vi "Cmd Get Parameter Properties (C).vi"(4 "error in (no error)":errorcluster, 6 "parameter index":variant, 7 "command reference":T4) -> (0 "error out":errorcluster, 1 "parameter properties":T1, 3 "command reference out":T4)   [LabVIEW 2017, in "NI_Database_API.lvlib"]
doc: "Gets properties of the object as determined by the inputs. This VI works for connections, commands, recordsets, columns, and parameters. Wire data to the reference input to determine the polymorphic instance to use or manually select the instance."
uses:
  <vilib>/addons/database/NI_Database_API.lvlib
  <vilib>/addons/database/Command.llb/Cmd ObjectReference.ctl
  <vilib>/addons/database/Command.llb/Cmd Parameter Properties.ctl
  <vilib>/addons/database/Auxilliary.llb/DB Tools DataTypes.ctl
  <vilib>/addons/database/Auxilliary.llb/DB Tools Parameter Dir.ctl
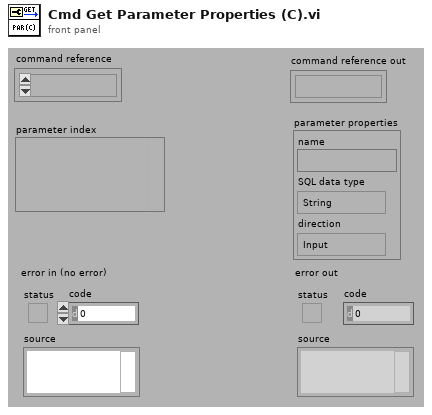
[diagram p1: front panel]
types:
  T1 = typedef "NI_Database_API.lvlib/Cmd Parameter Properties.ctl" = cluster{"name":string, "SQL data type":T2, "direction":T3}
  T2 = typedef "NI_Database_API.lvlib/DB Tools DataTypes.ctl" = enum16{"String", "Long (I32)", "Single (SGL)", "Double (DBL)", "Date/Time", "Binary"}
  T3 = typedef "NI_Database_API.lvlib/DB Tools Parameter Dir.ctl" = enum32{"Input", "Output", "Input/Output", "Return Value"}
  T4 = typedef "NI_Database_API.lvlib/Cmd ObjectReference.ctl" = refnum<k1>
  T5 = cluster{"Name":string, "data type":T2, "direction":T3}
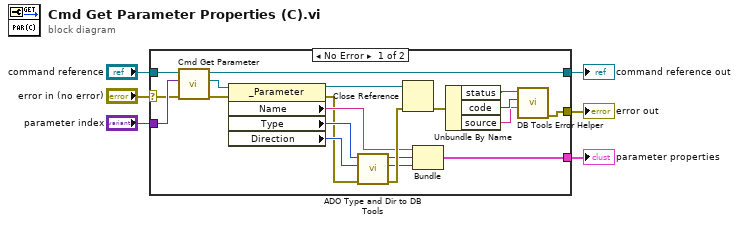
[diagram p0: block diagram]
diagram:
  n1 = case shown="No Error" "error in (no error)" {
    selector: "error in (no error)" -> [w7 w28]
    tunnel: [w24 _] -> w6
    tunnel: "command reference" -> [w17 w27]
    tunnel: "parameter index" -> [w16 _]
    tunnel: [w15 w27] -> w3
    tunnel: [w10 w28] -> w2
    frame No Error {
      n2 = call <vilib>:"Cmd Get Parameter.vi"("error in (no error)"=w7, "parameter index"=w16, "command reference"=w17) -> ("error out"=w13:errorcluster, "ADODB.Parameter"=w14:refnum<k7>, "command reference out"=w15:T4)  [unwired: 2 out]
      n3 = property class="_Parameter"(reference=w14, error in=w13) -> (reference out=w26:refnum<k7>, error out=w18:errorcluster, "Name"=w19:string, "Type"=w23:i32, "Direction"=w25:i32)
      n4 = call <vilib>:"ADO Type and Dir to DB Tools.vi"("error in (no error)"=w18, "ADO direction"=w25, "ADO type"=w23) -> ("error out"=w22:errorcluster, "direction"=w20:T3, "data type"=w21:T2)  [unwired: 2 out]
      n5 = Close Reference(reference=w26, error in (no error)=w22) -> (error out=w11:errorcluster)
      n6 = Bundle("Name"=w19, "data type"=w21, "direction"=w20) -> (w24:T5)  [unwired: 1 out]
      n7 = Unbundle By Name(w11) -> ("status"=w12:bool, "code"=w9:i32, "source"=w8:string)
      n8 = call <vilib>:"DB Tools Error Helper.vi"("source"=w8, "code"=w9, "status"=w12) -> ("error out"=w10:errorcluster)  [unwired: 1 in, 7 out]
    }
    frame Error {
    }
  }
  "command reference out" <- w3
  "error out" <- w2
  "parameter properties" <- w6
